vi "Midi_main.vi"(11 "hub":string) -> ()   [LabVIEW 2022 SP3]
panel:
  in  "Tab Control":T1(tab)
  in  "Test":bool
  in  "advertise":bool
  in  "Run":bool
  in  "note length (msec)":u8(slide)=104 scale=0.0..1000.0
  in  "Mapping formula":string="(sensor-40)/15+48"
  out "Converted note":string
  in  "Port":u16(ring) items=["A", "B", "C", "D", "E", "F"]
  in  "Sensor":u16(ring) items=["proximity", "light (color)", "light (reflected)", "force", "motor"]
  in  "BLE Name":string="something"
  out "current value":dbl(knob) scale=0.0..100.0
  in  "send":string
  in  "Read":bool
  out "sensor read":string
  out "Console":string
  out "Code":string
  out "advertising":bool
  out "python good":bool
  out "error out":errorcluster
  out "ble?":bool
  in  "done":bool
  # "1. Select your sensor and port\n2. Choose a BLE name and start advertising\n3. Connect on GarageBand (under settings/Advanced/Bluetooth )\n4.  Figure out your mapping formula\n5. Hit run"
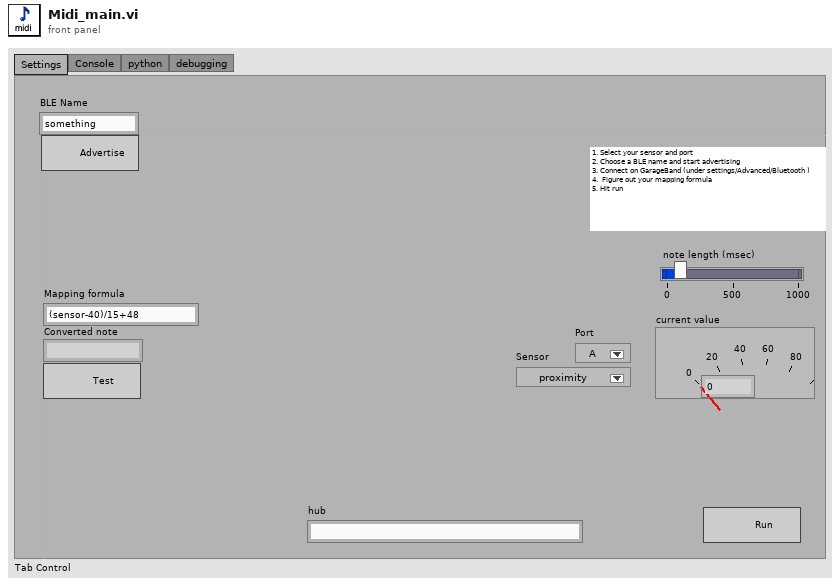
[diagram p1: front panel]
types:
  T1 = enum32{"Settings", "Console", "python", "debugging"}
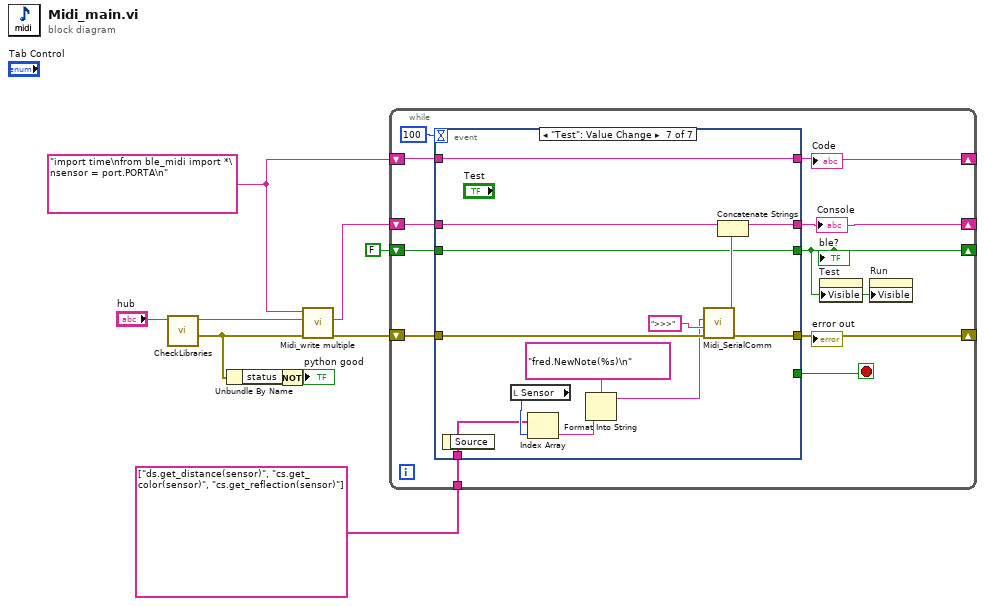
[diagram p0: block diagram]
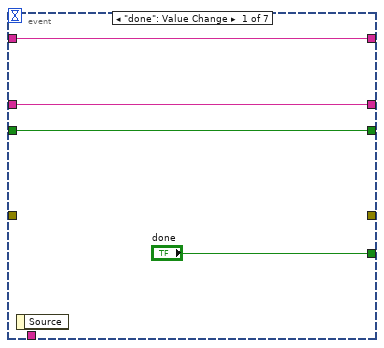
[diagram p2: hidden frame]
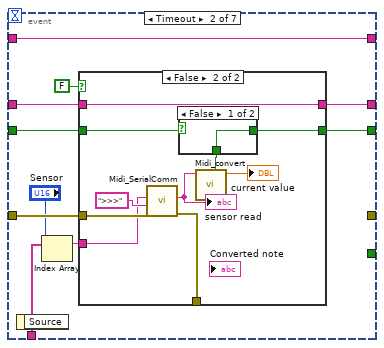
[diagram p3: hidden frame]
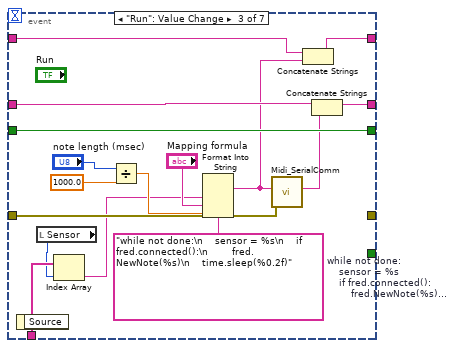
[diagram p6: hidden frame]
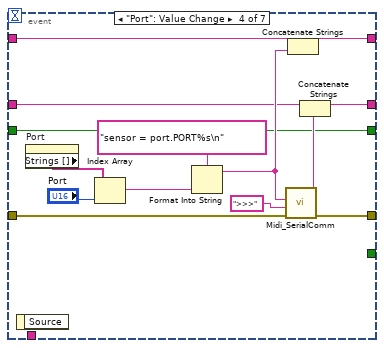
[diagram p7: hidden frame]
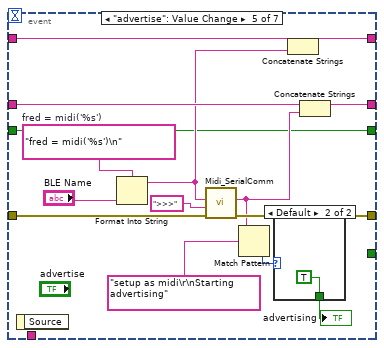
[diagram p8: hidden frame]
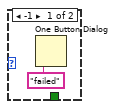
[diagram p9: hidden frame]
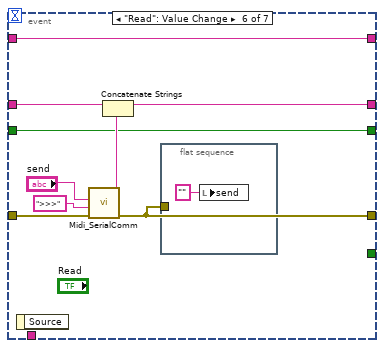
[diagram p10: hidden frame]
diagram:
  w3 = "import time\nfrom ble_midi import *\nsensor = port.PORTA\n"
  n1 = call "CheckLibraries.vi"("hub"="hub") -> ("error out"=w4:errorcluster, "console out"=w6:string)  [unwired: 9 in]
  n2 = Unbundle By Name(w4) -> ("status"=w9:bool)
  n3 = Not(x=w9) -> (.not. x?=→"python good":bool)
  n4 = call "Midi_write multiple.vi"("error in (no error)"=w4, "console in"=w6, "to write"=w3) -> ("error out"=w10:errorcluster, "console out"=w5:string)  [unwired: 7 in]
  n5 = while {
    shift-right: [w17] -> _
    shift-left: w5 -> [w18]
    shift-right: [w15] -> _
    shift-left: w3 -> [w16]
    shift-right: [w14] -> _
    shift-left: w10 -> [w21]
    shift-right: [w12] -> _
    shift-left: FALSE ("ble?") -> [w13]
    tunnel: string[] ["ds.get_distance(sensor)", "cs.get_color(sensor)", "cs.get_reflection(sensor)"] -> [w11]
    stop <- w20 stop-if-true
    n6 = event shown="[6] \"Test\": Value Change" {
      selector: _ -> [_ _ _ _ _ _ _]
      dyn-events: _ -> [_ _ _ _ _ _ _]
      timeout: 100 -> [_ _ _ _ _ _ _]
      tunnel: w21 -> [_ w35 w65 w74 w93 w104 w118]
      tunnel: ["done" _ _ _ _ _ _] -> w20
      tunnel: w18 -> [w24 w34 w64 w69 w89 w103 w117]
      tunnel: [w24 w33 w63 w67 w88 w101 w115] -> w17
      tunnel: [w23 w32 w53 w70 w90 w100 w114] -> w15
      tunnel: w16 -> [w23 w32 w55 w72 w91 w100 w114]
      tunnel: [_ _ _ w73 w92 w98 w113] -> w14
      tunnel: [w22 w31 w62 w66 w80 w97 w112] -> w12
      tunnel: w13 -> [w22 w30 w62 w66 w80 w97 w112]
      tunnel: w11 -> [_ w28 w52 _ _ _ w108]
      event "done": Value Change {
        n7 = event-data() -> ()  [unwired: 1 in, 1 out]
      }
      event Timeout {
        n8 = event-data() -> ()  [unwired: 1 in, 1 out]
        n9 = Index Array(array=w28, index="Sensor") -> (element=w26:string)
        n10 = case shown="False" FALSE {
          tunnel: w35 -> [_ w46]
          tunnel: w26 -> [_ w45]
          tunnel: w34 -> [w36 w42]
          tunnel: [w36 w42] -> w33
          tunnel: [_ w41] -> _
          tunnel: [w37 w40] -> w31
          tunnel: w30 -> [w37 w38]
          frame True {
          }
          frame False {
            n11 = call "Midi_SerialComm.vi"("error in (no error)"=w46, "wait for"=">>>", "To send"=w45) -> ("error out"=w41:errorcluster, "read"=w44:string)  [unwired: 7 in]
            "sensor read" <- w44
            n12 = call "Midi_convert.vi"("read"=w44) -> ("current value"=→"current value":dbl, "ble?"=w39:bool)  [unwired: 9 in]
            n13 = case shown="False" w38 {
              selector: w38 -> [_ w49]
              tunnel: [w48 w49] -> w40
              tunnel: w39 -> [w48 _]
              frame False {
              }
              frame True {
              }
            }
          }
        }
      }
      event "Run": Value Change {
        w56 = "while not done:\n    sensor = %s\n    if fred.connected():\n        fred.NewNote(%s)\n    time.sleep(%0.2f)"  # while not done:     sensor = %s     if fred.connected():         fred.NewNote(%s)     time.sleep(%0.2f)
        n14 = event-data() -> ()  [unwired: 1 in, 1 out]
        n15 = local read "Sensor"() -> (w51:u16)
        n16 = Index Array(array=w52, index=w51) -> (element=w50:string)
        n17 = Divide(x="note length (msec)", y=1000.0) -> (x/y=w60:dbl)
        n18 = Format Into String(format string=w56, w50, "Mapping formula", w60) -> (resulting string=w54:string)  [unwired: 2 in, 1 out]
        n19 = call "Midi_SerialComm.vi"("error in (no error)"=w65, "To send"=w54) -> ("read"=w61:string)  [unwired: 8 in, 1 out]
        n20 = Concatenate Strings(w55, w54) -> (w53:string)
        n21 = Concatenate Strings(w64, w61) -> (w63:string)
      }
      event "Port": Value Change {
        n22 = event-data() -> ()  [unwired: 1 in, 1 out]
        n23 = property on="Port" class="Ring (strict)"() -> ("Strings []"=w77:string[])  [unwired: 2 in, 2 out]
        n24 = Index Array(array=w77, index="Port") -> (element=w79:string)
        n25 = Format Into String(format string="sensor = port.PORT%s\n", w79) -> (resulting string=w71:string)  [unwired: 2 in, 1 out]
        n26 = call "Midi_SerialComm.vi"("error in (no error)"=w74, "wait for"=">>>", "To send"=w71) -> ("error out"=w73:errorcluster, "read"=w68:string)  [unwired: 7 in]
        n27 = Concatenate Strings(w72, w71) -> (w70:string)
        n28 = Concatenate Strings(w69, w68) -> (w67:string)
      }
      event "advertise": Value Change {
        w86 = "fred = midi('%s')\n"  # fred = midi('%s')
        n29 = event-data() -> ()  [unwired: 1 in, 1 out]
        n30 = Format Into String(format string=w86, "BLE Name") -> (resulting string=w85:string)  [unwired: 2 in, 1 out]
        n31 = call "Midi_SerialComm.vi"("error in (no error)"=w93, "wait for"=">>>", "To send"=w85) -> ("error out"=w92:errorcluster, "read"=w84:string)  [unwired: 7 in]
        n32 = Match Pattern(string=w84, regular expression="setup as midi\r\nStarting advertising") -> (offset past match=w82:i32)  [unwired: 1 in, 3 out]
        n33 = case shown="Default" w82 {
          tunnel: [_ TRUE] -> w81
          frame -1 {
            n34 = One Button Dialog(message="failed") -> ()  [unwired: 1 in, 1 out]
          }
          frame Default {
          }
        }
        "advertising" <- w81
        n35 = Concatenate Strings(w91, w85) -> (w90:string)
        n36 = Concatenate Strings(w89, w84) -> (w88:string)
      }
      event "Read": Value Change {
        n37 = event-data() -> ()  [unwired: 1 in, 1 out]
        n38 = call "Midi_SerialComm.vi"("error in (no error)"=w104, "wait for"=">>>", "To send"="send") -> ("error out"=w98:errorcluster, "read"=w102:string)  [unwired: 7 in]
        n39 = Concatenate Strings(w103, w102) -> (w101:string)
        n40 = flat-sequence {
          tunnel: w98 -> [_]
          frame #0 {
            n41 = local write "send"("" ("send")) -> ()
          }
        }
      }
      event "Test": Value Change {
        n42 = event-data() -> ()  [unwired: 1 in, 1 out]
        n43 = local read "Sensor"() -> (w109:u16)
        n44 = Index Array(array=w108, index=w109) -> (element=w107:string)
        n45 = Format Into String(format string="fred.NewNote(%s)\n", w107) -> (resulting string=w110:string)  [unwired: 2 in, 1 out]
        n46 = call "Midi_SerialComm.vi"("error in (no error)"=w118, "wait for"=">>>", "To send"=w110) -> ("error out"=w113:errorcluster, "read"=w116:string)  [unwired: 7 in]
        n47 = Concatenate Strings(w117, w116) -> (w115:string)
      }
    }
    "Console" <- w17
    "Code" <- w15
    "error out" <- w14
    "ble?" <- w12
    n48 = property on="Test" class="Bool"("Visible"=w12) -> ()  [unwired: 2 in, 2 out]
    n49 = property on="Run" class="Bool"("Visible"=w12) -> ()  [unwired: 2 in, 2 out]
  }
